vi "SSL Detection Balls Delete Invalids with State and Cov.vi"(5 "Now":timestamp, 7 "Life Time":dbl=1.0, 11 "Array":T3(array[cluster])=[{"Detection Ball"={"x"=10.0, "area"=0, "confidence"=0.0, "y"=10.0, "z"=0.0, "pixel_x"=0.0, "pixel_y"=0.0, "Valid"=FALSE, "Time Stamp"=timestamp(0 s since 1904-01-01)}, "Pose"=[], "Pk|k"=[]}, {"Detection Ball"={"x"=20.0, "area"=0, "confidence"=0.0, "y"=20.0, "z"=0.0, "pixel_x"=0.0, "pixel_y"=0.0, "Valid"=FALSE, "Time Stamp"=timestamp(0 s since 1904-01-01)}, "Pose"=[], "Pk|k"=[]}]) -> (2 "Array 2":T3(array[cluster]), 3 "Balls Out":T1[](array[typedef]))   [LabVIEW 2016]
uses:
  SSL Detection Ball.ctl
  <vilib>/Analysis/Matrix/Datatypes/RealMatrix.ctl
  <vilib>/Analysis/Matrix/NI_Matrix.lvlib
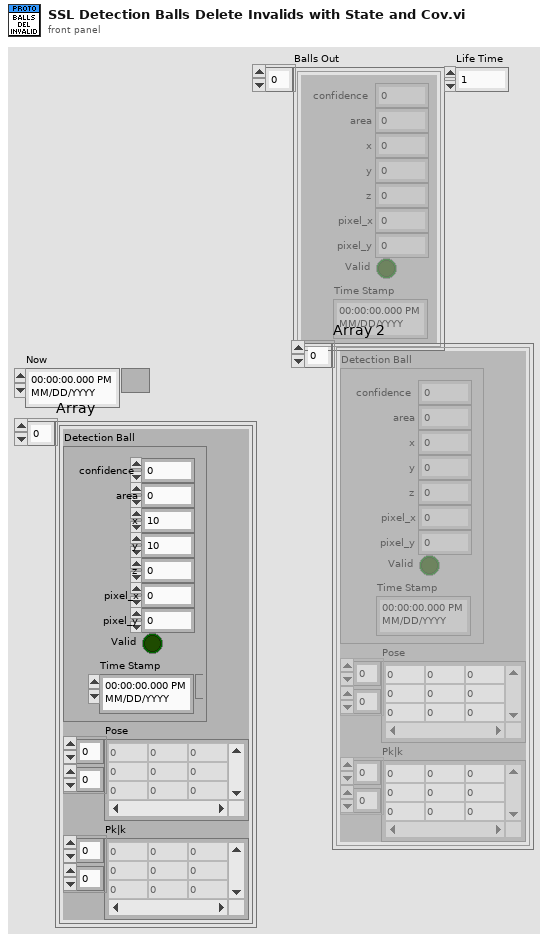
[diagram p1: front panel]
types:
  T1 = typedef "SSL Detection Ball.ctl" = cluster{"x":sgl, "area":u32, "confidence":sgl, "y":sgl, "z":sgl, "pixel_x":sgl, "pixel_y":sgl, "Valid":bool, "Time Stamp":timestamp}
  T2 = typedef "NI_Matrix.lvlib/RealMatrix.ctl" = dbl[][]
  T3 = cluster{"Detection Ball":T1, "Pose":T2, "Pk|k":T2}[]
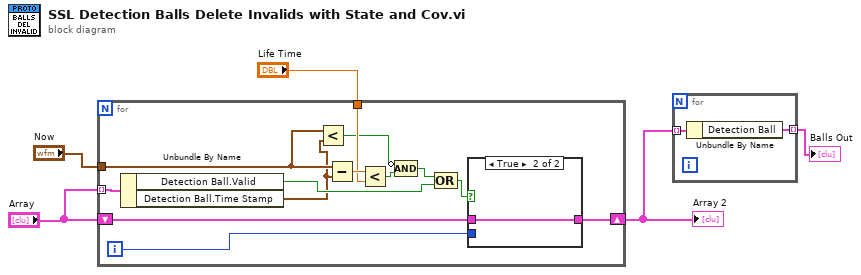
[diagram p0: block diagram]
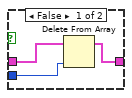
[diagram p2: hidden frame]
diagram:
  n1 = for {
    tunnel: "Array" -> [w18] mode=indexing
    shift-right: [w15] -> w2
    shift-left: "Array" -> [w17]
    tunnel: "Now" -> [w10]
    tunnel: "Life Time" -> [w13]
    i -> [w16]
    n2 = Unbundle By Name(w18) -> ("Detection Ball.Valid"=w12:bool, "Detection Ball.Time Stamp"=w9:timestamp)
    n3 = Less?(x=w10, y=w9) -> (x < y?=w7:bool)
    n4 = Subtract(x=w10, y=w9) -> (x-y=w14:dbl)
    n5 = Less?(x=w14, y=w13) -> (x < y?=w8:bool)
    n6 = Compound Arithmetic op=AND(invert w7, w8) -> (w6:bool)
    n7 = Compound Arithmetic op=OR(w6, w12) -> (w11:bool)
    n8 = case shown="True" w11 {
      tunnel: w17 -> [w21 w22]
      tunnel: w16 -> [w20 _]
      tunnel: [w19 w22] -> w15
      frame False {
        n9 = Delete From Array(array=w21, index=w20) -> (array with subset deleted=w19:T3)  [unwired: 1 in, 1 out]
      }
      frame True {
      }
    }
  }
  "Array 2" <- w2
  n10 = for {
    tunnel: w2 -> [w24] mode=indexing
    tunnel: [w23] -> w1 mode=indexing
    n11 = Unbundle By Name(w24) -> ("Detection Ball"=w23:T1)
  }
  "Balls Out" <- w1
